vi "niP2P Disable Peer to Peer Stream.vi"(0 "stream session":refnum<k20>, 11 "error in (no error)":errorcluster) -> (4 "stream session out":refnum<k20>, 15 "error out":errorcluster)   [LabVIEW 2010]
doc: "Immediately disables a stream without flushing data from the writer. Any existing data in the writer is lost. To avoid data loss and guarantee all existing data in the writer is flushed to the reader before disabling the stream, use the niP2P Flush And Disable Peer to Peer Stream VI."
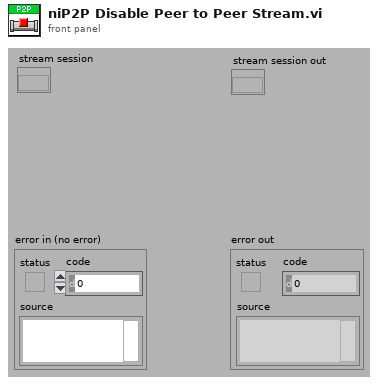
[diagram p1: front panel]
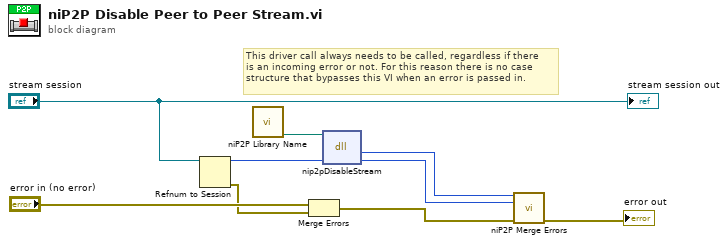
[diagram p0: block diagram]
diagram:
  # "This driver call always needs to be called, regardless if there\nis an incoming error or not. For this reason there is no case\nstructure that bypasses this VI when an error is passed in."
  n1 = Refnum to Session(7:"stream session") -> (0:w2:errorcluster, 3:w9:u64)  [unwired: 1 in]
  n2 = call <vilib>:"niP2P Library Name.vi"() -> ("nip2p libname"=w1:path)  [unwired: 10 in]
  n3 = Merge Errors("error in (no error)", w2) -> (w4:errorcluster)
  n4 = dll-call lib="?" fn="nip2pDisableStream"(path in=w1, "streamHandle"=w9) -> ("return type"=w7:i32, "streamHandle"=w5:u32)  [unwired: 2 in, 2 out]
  n5 = call <vilib>:"niP2P Merge Errors.vi"("error code"=w7, "stream handle (0)"=w5, "error in"=w4) -> ("error out"=→"error out":errorcluster)  [unwired: 12 in]
  "stream session out" <- "stream session"
